vi "AlliGator Is Decay Valid.vi"(8 "Error In":errorcluster, 10 "Plot Name":string, 11 "Decay":cluster{"t Array":dbl[], "Value Array":dbl[]}) -> (0 "Error Out":errorcluster, 1 "Is Valid?":bool, 2 "Message":string, 3 "Decay (dup)":cluster{"t Array":dbl[], "Value Array":dbl[]})   [LabVIEW 2021, in "AlliGator Decay Fit.lvlib"]
doc: "Checks whether the input <B>Decay</B> is valid, i.e. is non-zero, does not contain NaN and has more than one element."
uses:
  AlliGator Decay Fit.lvlib
  <vilib>/Utility/error.llb/Error Cluster From Error Code.vi
  <vilib>/ErrorRing/Error Ring.xnode
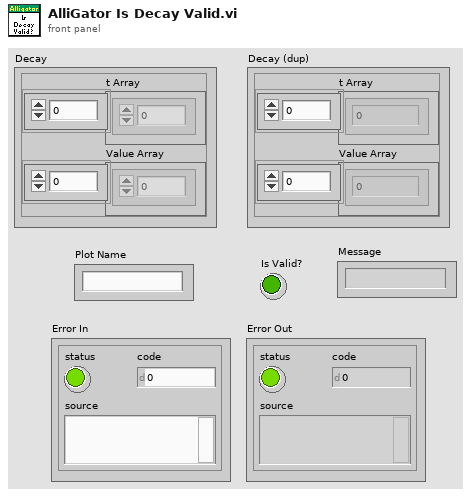
[diagram p1: front panel]
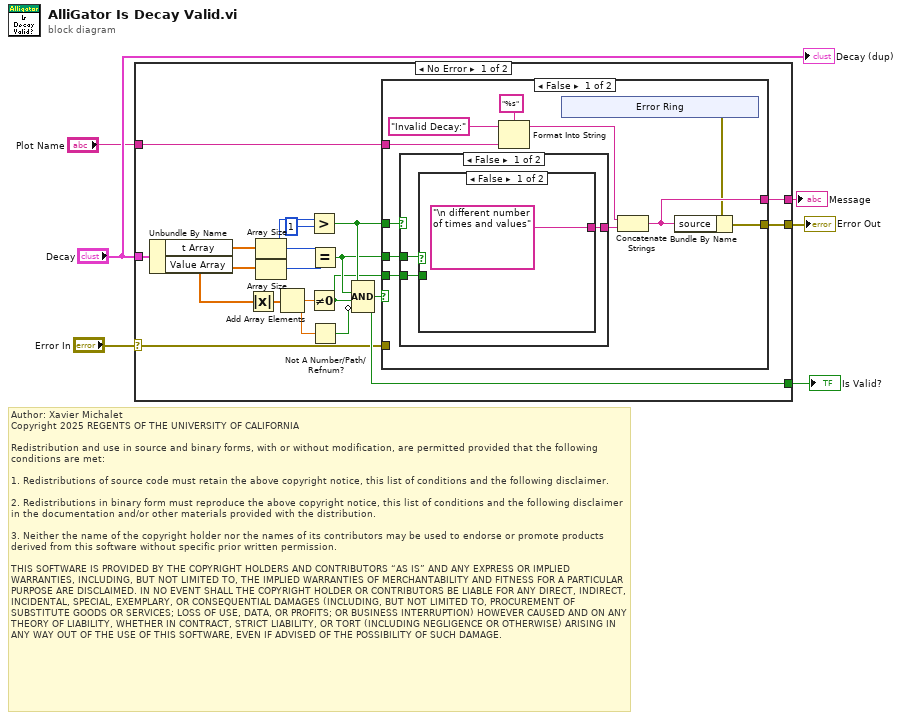
[diagram p0: block diagram]
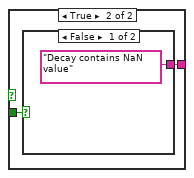
[diagram p2: hidden frame]
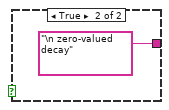
[diagram p3: hidden frame]
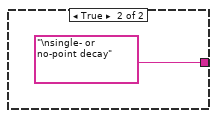
[diagram p4: hidden frame]
diagram:
  # "Author: Xavier Michalet\nCopyright 2025 REGENTS OF THE UNIVERSITY OF CALIFORNIA\n\nRedistribution and use in source and binary forms, with or without modification, are permitted provided that the following conditions are met:\n\n1. Redistributions of source code must retain the above copyright notice, this list of conditions and the following disclaimer.\n\n2. Redistributions in binary form must reproduce the above copyright notice, this list of conditions and the following disclaimer in the documentation and/or other materials provided with the distribution.\n\n3. Neither the name of the copyright holder nor the names of its contributors may be used to endorse or promote products derived from this software without specific prior written permission.\n\nTHIS SOFTWARE IS PROVIDED BY THE COPYRIGHT HOLDERS AND CONTRIBUTORS “AS IS” AND ANY EXPRESS OR IMPLIED WARRANTIES, INCLUDING, BUT NOT LIMITED TO, THE IMPLIED WARRANTIES OF MERCHANTABILITY AND FITNESS FOR A PARTICULAR PURPOSE ARE DISCLAIMED. IN NO EVENT SHALL THE COPYRIGHT HOLDER OR CONTRIBUTORS BE LIABLE FOR ANY DIRECT, INDIRECT, INCIDENTAL, SPECIAL, EXEMPLARY, OR CONSEQUENTIAL DAMAGES (INCLUDING, BUT NOT LIMITED TO, PROCUREMENT OF SUBSTITUTE GOODS OR SERVICES; LOSS OF USE, DATA, OR PROFITS; OR BUSINESS INTERRUPTION) HOWEVER CAUSED AND ON ANY THEORY OF LIABILITY, WHETHER IN CONTRACT, STRICT LIABILITY, OR TORT (INCLUDING NEGLIGENCE OR OTHERWISE) ARISING IN ANY WAY OUT OF THE USE OF THIS SOFTWARE, EVEN IF ADVISED OF THE POSSIBILITY OF SUCH DAMAGE."
  n1 = case shown="No Error" "Error In" {
    selector: "Error In" -> [w8 w49]
    tunnel: [w10 _] -> w6
    tunnel: "Decay" -> [w23 _]
    tunnel: [w13 _] -> w4
    tunnel: "Plot Name" -> [w14 _]
    tunnel: [w9 w49] -> w1
    frame No Error {
      n2 = Unbundle By Name(w23) -> ("t Array"=w22:dbl[], "Value Array"=w18:dbl[])
      n3 = Absolute Value(x=w18) -> (abs(x)=w17:dbl[])
      n4 = Array Size(array=w22) -> (size(s)=w20:i32)
      n5 = Array Size(array=w18) -> (size(s)=w21:i32)
      n6 = Add Array Elements(numeric array=w17) -> (sum=w12:dbl)
      n7 = Greater?(x=w20, y=1) -> (0:w16:bool)
      n8 = Not Equal To 0?(x=w12) -> (x != 0?=w7:bool)
      n9 = Equal?(x=w20, y=w21) -> (x = y?=w15:bool)
      n10 = Not A Number/Path/Refnum?(number/path/refnum=w12) -> (NaN/Path/Refnum?=w11:bool)
      n11 = Compound Arithmetic op=AND(w16, w15, w7, invert w11) -> (w10:bool)
      n12 = case shown="False" w10 {
        tunnel: w16 -> [w34 _]
        tunnel: w15 -> [w33 _]
        tunnel: w14 -> [w29 _]
        tunnel: [w27 _] -> w13
        tunnel: [w26 w48] -> w9
        tunnel: w8 -> [_ w48]
        tunnel: w7 -> [w24 _]
        frame False {
          n13 = case shown="False" w34 {
            tunnel: w33 -> [w40 _]
            tunnel: [w41 "\nsingle- or no-point decay" ("Message")] -> w32
            tunnel: w24 -> [w39 _]
            frame False {
              n14 = case shown="False" w40 {
                tunnel: ["\n different number of times and values" ("Message") w44] -> w41
                tunnel: w39 -> [_ w43]
                frame False {
                }
                frame True {
                  n15 = case shown="False" w43 {
                    tunnel: ["Decay contains NaN value" ("Message") "\n zero-valued decay" ("Message")] -> w44
                    frame False {
                    }
                    frame True {
                    }
                  }
                }
              }
            }
            frame True {
            }
          }
          n16 = Format Into String(format string="%s", initial string="Invalid Decay:", w29) -> (resulting string=w28:string)  [unwired: 1 in, 1 out]
          n17 = xnode "Error Ring"() -> ("error out"=w25:errorcluster)
          n18 = Concatenate Strings(w28, w32) -> (w27:string)
          n19 = Bundle By Name(cluster=w25, "source"=w27) -> (w26:errorcluster)
        }
        frame True {
        }
      }
    }
    frame Error {
    }
  }
  "Error Out" <- w1
  "Is Valid?" <- w6
  "Message" <- w4
  "Decay (dup)" <- "Decay"
